vi "Format to Internal Technique Parameters.vi"(8 "error in (no error)":errorcluster, 9 "Technique Parameters (Typedefs)":variant, 10 "Technique":T1, 11 "Potentiostat Galvanostat in":refnum<class "Potentiostat Galvanostat.lvclass">) -> (0 "error out":errorcluster, 2 "Internal Technique Parameters":variant, 3 "Potentiostat Galvanostat out":refnum<class "Potentiostat Galvanostat.lvclass">)   [LabVIEW 2018, in "Potentiostat Galvanostat.lvclass"]
uses:
  Potentiostat Galvanostat.lvclass
  Controls/Technique List.ctl
  Controls/Error Codes.ctl
  Potentiostat Galvanostat.lvclass/Potentiostat Galvanostat.ctl
  Controls/OCV Parameters.ctl
  Controls/OCV Internal Parameters.ctl
  Controls/CV Parameters.ctl
  Controls/CV Internal Parameters.ctl
  Controls/CA Parameters.ctl
  Controls/CA Internal Parameters.ctl
  Controls/CP Parameters.ctl
  Controls/CP Internal Parameters.ctl
  Controls/PEIS Parameters.ctl
  Controls/PEIS Internal Parameters.ctl
  Controls/GEIS Parameters.ctl
  Controls/GEIS Internal Parameters.ctl
  BL_GetErrorMsg.vi
  <vilib>/Utility/error.llb/Error Cluster From Error Code.vi
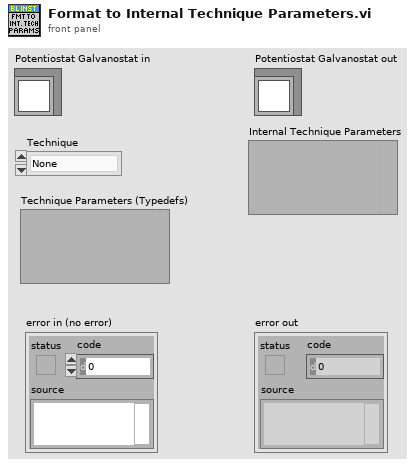
[diagram p1: front panel]
types:
  T1 = typedef "Potentiostat Galvanostat.lvclass/Technique List.ctl" = enum16{"None", "ocv", "cv", "biovscan", "ca", "cp", "iscan", "vscan", "lasv", "load", "pow", "peis", "geis", "seisp", "seisg", "dpv", "swv", "npv", "mpv", "dnpv", "dpa", "evt", "lp", "gc", "cpp", "pdp", "psp", "zra", "ircmp", "pzir", "gzir", "loop", "TO", "TI", "TOS", "vscanlimit", "iscanlimit", "mp", "casp", "casg", "calimit", "cplimit"}
  T2 = typedef "Potentiostat Galvanostat.lvclass/OCV Parameters.ctl" = cluster{"Rest duration (s)":sgl, "Record every dE (V)":sgl, "Record every dT (s)":sgl, "Ewe range":u16, "CE to ground Mode":u16}
  T3 = typedef "Potentiostat Galvanostat.lvclass/OCV Internal Parameters.ctl" = cluster{"Rest_time_T":sgl, "Record_every_dE":sgl, "Record_every_dT":sgl, "E_Range":u16, "em":u16, "ce":u16, "tb":sgl}
  T4 = typedef "Potentiostat Galvanostat.lvclass/CV Parameters.ctl" = cluster{"Ei Params":cluster{"Current step vs initial one (Ei)":bool, "Voltage step (V) (Ei)":sgl, "slew rate array (mV/s) (Ei)":sgl}, "E1 Params":cluster{"Current step vs initial one (E1)":bool, "Voltage step (V) (E1)":sgl, "slew rate array (mV/s) (E1)":sgl}, "E2 Params":cluster{"Current step vs initial one (E2)":bool, "Voltage step (V) (E2)":sgl, "slew rate array (mV/s) (E2)":sgl}, "Ef Params":cluster{"Current step vs initial one (Ef)":bool, "Voltage step (V) (Ef)":sgl, "slew rate array (mV/s) (Ef)":sgl}, "Number of cycle":i32, "recording on dE (V)":sgl, "average every dE":bool, "Begin step accumulation (1 = 100% of step)":sgl, "End step accumulation ( 1 = 100% of step)":sgl, "I range":u16, "Bandwidth":u16, "Ewe range":u16, "CE to ground Mode":u16}
  T5 = typedef "Potentiostat Galvanostat.lvclass/CV Internal Parameters.ctl" = cluster{"Voltage_steps":cluster{"vs_initial":bool, "Voltage_step":sgl, "Scan_Rate":sgl}[], "N_Cycles":i32, "Record_every_dE":sgl, "Average_over_dE":bool, "Begin_measuring_I":sgl, "End_measuring_I":sgl, "I_Range":u16, "E_Range":u16, "Bandwidth":u16, "em":u16, "ce":u16, "Scan_number":u16, "tb":sgl}
  T6 = typedef "Potentiostat Galvanostat.lvclass/CA Parameters.ctl" = cluster{"Voltage Steps":cluster{"Voltage step vs initial one":bool, "Voltage step (V)":sgl, "Duration step (s)":sgl}[], "No. of steps":i32, "Record every dt (s)":sgl, "Record every dI (A)":sgl, "No. of times\ntechnique is repeated":i32, "I range":u16, "Ewe range":u16, "Bandwidth":u16, "CE to ground Mode":u16}
  T7 = typedef "Potentiostat Galvanostat.lvclass/CA Internal Parameters.ctl" = cluster{"tb":sgl, "Voltage_steps":cluster{"vs_initial":bool, "Voltage_step":sgl, "Duration_step":sgl}[], "Step_number":i32, "N_Cycles":i32, "Record_every_dI":sgl, "Record_every_dT":sgl, "I_Range":u16, "E_Range":u16, "Bandwidth":u16, "em":u16, "ce":u16}
  T8 = typedef "Potentiostat Galvanostat.lvclass/CP Parameters.ctl" = cluster{"Current Steps":cluster{"Current step vs initial\none":bool, "Current step (A)":sgl, "Duration step (s)":sgl}[], "No. of steps":i32, "Record every dt (s)":sgl, "Record every dE (V)":sgl, "No. of times\ntechnique is repeated":i32, "I range":u16, "Ewe range":u16, "Bandwidth":u16, "CE to ground Mode":u16}
  T9 = typedef "Potentiostat Galvanostat.lvclass/CP Internal Parameters.ctl" = cluster{"Current_steps":cluster{"vs_initial":bool, "Current_step":sgl, "Duration_step":sgl}[], "Step_number":i32, "N_Cycles":i32, "Record_every_dE":sgl, "Record_every_dT":sgl, "I_Range":u16, "E_Range":u16, "Bandwidth":u16, "em":u16, "ce":u16, "tb":sgl}
  T10 = typedef "Potentiostat Galvanostat.lvclass/PEIS Parameters.ctl" = cluster{"Step duration (s)":sgl, "Record every dI (A)":sgl, "Record every dt (s)":sgl, "Initial voltage step (V)":sgl, "Voltage step vs initial one":bool, "Initial frequency (Hz)":sgl, "sweep linear/logarithmic":bool, "Number of frequencies":i32, "Final frequency (Hz)":sgl, "Sine amplitude (V)":sgl, "No. of repeat times":i32, "No. of period to wait\nbefore each frequency":sgl, "Non-stationary correction":bool, "I Range":u16, "Bandwidth":u16, "CE to ground Mode":u16}
  T11 = typedef "Potentiostat Galvanostat.lvclass/PEIS Internal Parameters.ctl" = cluster{"Step_number":i32, "Initial_Voltage_step":sgl, "vs_initial":bool, "Final_Voltage_step":sgl, "vs_final":bool, "Duration_step":sgl, "Record_every_dI":sgl, "Record_every_dT":sgl, "Initial_frequency":sgl, "sweep":bool, "Final_frequency":sgl, "Frequency_number":i32, "Amplitude_Voltage":sgl, "Wait_for_steady":sgl, "Average_N_times":i32, "Correction":bool, "I_Range":u16, "Bandwidth":u16, "em":u16, "ce":u16}
  T12 = typedef "Potentiostat Galvanostat.lvclass/GEIS Parameters.ctl" = cluster{"Initial frequency (Hz)":sgl, "sweep linear/logarithmic":bool, "Number of frequencies":i32, "Final frequency (Hz)":sgl, "Sine amplitude (A)":sgl, "No. of repeat times":i32, "No. of period to wait\nbefore each frequency":sgl, "Non-stationary correction":bool, "I Range":u16, "Bandwidth":u16, "CE to ground Mode":u16, "Step duration (s)":sgl, "Record every dE (V)":sgl, "Record every dt (s)":sgl, "Initial current step (A)":sgl, "Current step vs initial one":bool}
  T13 = typedef "Potentiostat Galvanostat.lvclass/GEIS Internal Parameters.ctl" = cluster{"Step_number":i32, "Initial_Current_step":sgl, "vs_initial ":bool, "Final_Current_step":sgl, "vs_final":bool, "Duration_step":sgl, "Record_every_dE":sgl, "Record_every_dT":sgl, "Initial_frequency":sgl, "sweep":bool, "Final_frequency":sgl, "Frequency_number":i32, "Amplitude_Current":sgl, "Wait_for_steady":sgl, "Average_N_times":i32, "Correction":bool, "I_Range":u16, "Bandwidth":u16, "em":u16, "ce":u16}
  T14 = typedef "Potentiostat Galvanostat.lvclass/Error Codes.ctl" = i32
  T15 = cluster{"Current step vs initial one (Ei)":bool, "Voltage step (V) (Ei)":sgl, "slew rate array (mV/s) (Ei)":sgl}
  T16 = cluster{"Current step vs initial one (E1)":bool, "Voltage step (V) (E1)":sgl, "slew rate array (mV/s) (E1)":sgl}
  T17 = cluster{"Current step vs initial one (E2)":bool, "Voltage step (V) (E2)":sgl, "slew rate array (mV/s) (E2)":sgl}
  T18 = cluster{"Current step vs initial one (Ef)":bool, "Voltage step (V) (Ef)":sgl, "slew rate array (mV/s) (Ef)":sgl}
  T19 = cluster{"Current step vs initial one (Ef)":bool, "Voltage step (V) (Ef)":sgl, "slew rate array (mV/s) (Ef)":sgl}[]
  T20 = cluster{"Voltage step vs initial one":bool, "Voltage step (V)":sgl, "Duration step (s)":sgl}[]
  T21 = cluster{"Current step vs initial\none":bool, "Current step (A)":sgl, "Duration step (s)":sgl}[]
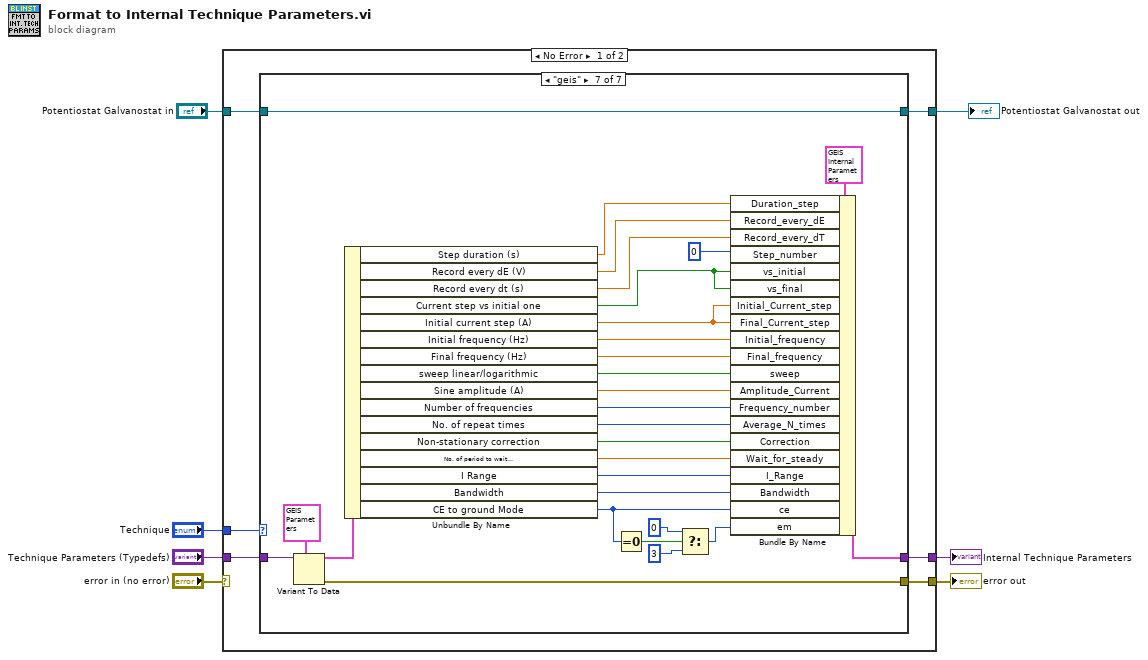
[diagram p0: block diagram]
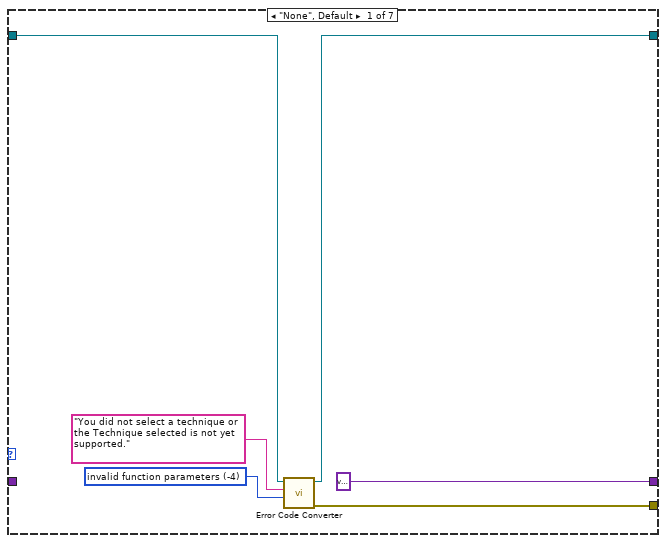
[diagram p2: hidden frame]
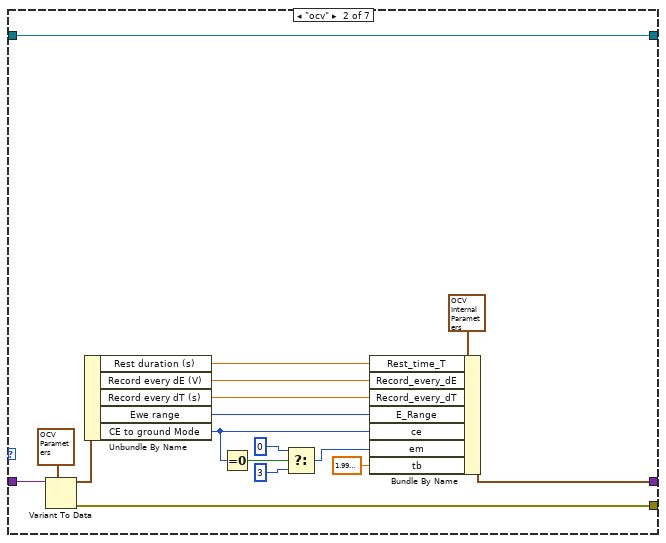
[diagram p3: hidden frame]
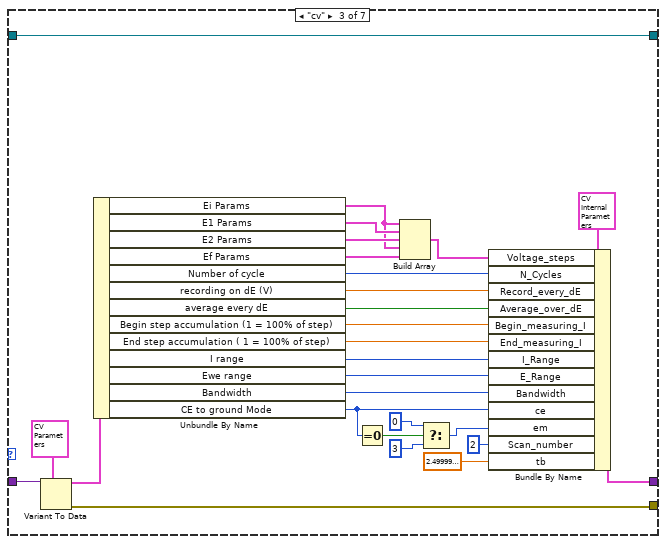
[diagram p4: hidden frame]
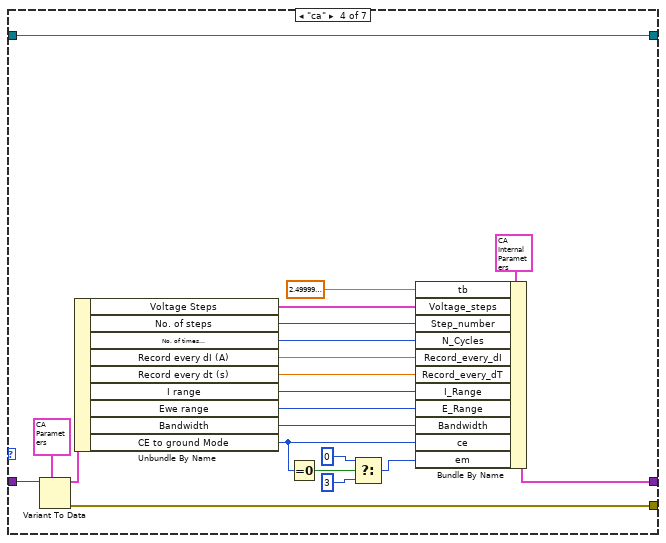
[diagram p5: hidden frame]
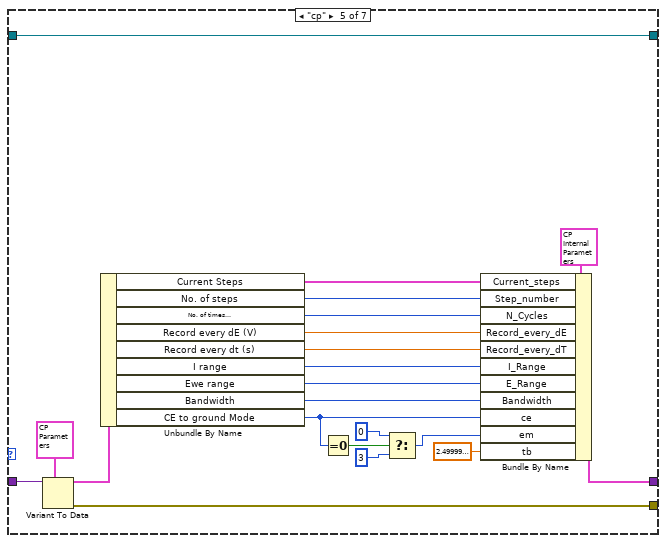
[diagram p6: hidden frame]
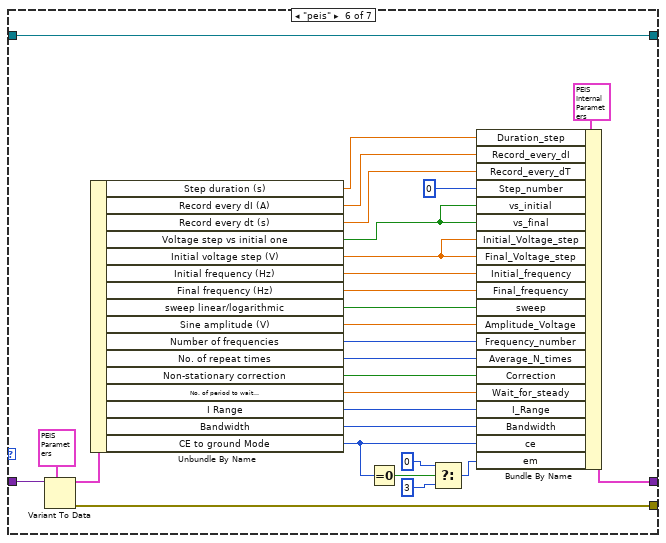
[diagram p7: hidden frame]
diagram:
  n1 = case shown="No Error" "error in (no error)" {
    selector: "error in (no error)" -> [_ w163]
    tunnel: "Technique" -> [w13 _]
    tunnel: "Technique Parameters (Typedefs)" -> [w12 _]
    tunnel: "Potentiostat Galvanostat in" -> [w11 w162]
    tunnel: [w10 w162] -> w4
    tunnel: [w9 w163] -> w3
    tunnel: [w8 _] -> w1
    frame No Error {
      n2 = case shown="\"geis\"" w13 {
        tunnel: w12 -> [_ w23 w39 w68 w87 w114 w141]
        tunnel: w11 -> [w17 w20 w63 w66 w105 w133 w161]
        tunnel: [w16 w20 w63 w66 w105 w133 w161] -> w10
        tunnel: [w14 w22 w38 w65 w86 w113 w140] -> w9
        tunnel: [variant ("Variant") w21 w37 w64 w85 w112 w139] -> w8
        frame "None", Default {
          w19 = T14 -4 items=["No Error"=0, "no instrument connected"=-1, "connection in progress"=-2, "selected channel(s) unplugged"=-3, "invalid function parameters"=-4, "selected file does not exist"=-5, "function failed"=-6, "no channel selected"=-7, "invalid instrument configuration"=-8, "EC-Lab firmware loaded on the instrument"=-9, "library not correctly loaded in memory"=-10, "USB library not correctly loaded in memory"=-11, "function of the library already in progress"=-12, "selected channel(s) already used"=-13, "device not allowed"=-14, "Invalid update function parameters"=-15, "internal instrument communication failed"=-101, "too many data to transfer from the instrument (device error)"=-102, "selected channel(s) unplugged (device error)"=-103, "instrument response error"=-104, "invalid message size"=-105] ("Error Code")
          n3 = call "Error Code Converter.vi"("Error Code"=w19, "Additional Description"="You did not select a technique or the Technique selected is not yet supported.", "Potentiostat Galvanostat in"=w17) -> ("error out"=w14:errorcluster, "Potentiostat Galvanostat out"=w16:refnum<class "Potentiostat Galvanostat.lvclass">)  [unwired: 7 in]
        }
        frame "ocv" {
          n4 = Variant To Data(type=T2 {"Rest duration (s)"=1.0, "Record every dE (V)"=0.01, "Record every dT (s)"=0.01, "Ewe range"=3, "CE to ground Mode"=0} ("OCV Parameters"), Variant=w23) -> (data=w25:T2, error out=w22:errorcluster)  [unwired: 1 in]
          n5 = Unbundle By Name(w25) -> ("Rest duration (s)"=w35:sgl, "Record every dE (V)"=w34:sgl, "Record every dT (s)"=w33:sgl, "Ewe range"=w32:u16, "CE to ground Mode"=w27:u16)
          n6 = Equal To 0?(x=w27) -> (x = 0?=w30:bool)
          n7 = Select(t=u16 0, s=w30, f=u16 3) -> (s? t:f=w26:u16)
          n8 = Bundle By Name(cluster=T3 {"Rest_time_T"=1.0, "Record_every_dE"=0.01, "Record_every_dT"=0.01, "E_Range"=3, "em"=1, "ce"=0, "tb"=2e-05} ("OCV Parameters"), "Rest_time_T"=w35, "Record_every_dE"=w34, "Record_every_dT"=w33, "E_Range"=w32, "ce"=w27, "em"=w26, "tb"=sgl 2e-05) -> (w21:T3)
        }
        frame "cv" {
          n9 = Variant To Data(type=T4 {"Ei Params"={"Current step vs initial one (Ei)"=TRUE, "Voltage step (V) (Ei)"=0.0, "slew rate array (mV/s) (Ei)"=0.1}, "E1 Params"={"Current step vs initial one (E1)"=FALSE, "Voltage step (V) (E1)"=0.1, "slew rate array (mV/s) (E1)"=0.1}, "E2 Params"={"Current step vs initial one (E2)"=FALSE, "Voltage step (V) (E2)"=-0.2, "slew rate array (mV/s) (E2)"=0.1}, "Ef Params"={"Current step vs initial one (Ef)"=TRUE, "Voltage step (V) (Ef)"=0.0, "slew rate array (mV/s) (Ef)"=0.1}, "Number of cycle"=1, "recording on dE (V)"=0.01, "average every dE"=TRUE, "Begin step accumulation (1 = 100% of step)"=0.5, "End step accumulation ( 1 = 100% of step)"=0.75, "I range"=12, "Bandwidth"=5, "Ewe range"=3, "CE to ground Mode"=0} ("CV Parameters"), Variant=w39) -> (data=w40:T4, error out=w38:errorcluster)  [unwired: 1 in]
          n10 = Unbundle By Name(w40) -> ("Ei Params"=w45:T15, "E1 Params"=w47:T16, "E2 Params"=w46:T17, "Ef Params"=w44:T18, "Number of cycle"=w61:i32, "recording on dE (V)"=w60:sgl, "average every dE"=w59:bool, "Begin step accumulation (1 = 100% of step)"=w58:sgl, "End step accumulation ( 1 = 100% of step)"=w57:sgl, "I range"=w56:u16, "Ewe range"=w55:u16, "Bandwidth"=w54:u16, "CE to ground Mode"=w50:u16)
          n11 = Equal To 0?(x=w50) -> (x = 0?=w53:bool)
          n12 = Build Array(w45, w47, w46, w45, w44) -> (w43:T19)
          n13 = Select(t=u16 0, s=w53, f=u16 3) -> (s? t:f=w49:u16)
          n14 = Bundle By Name(cluster=T5 {"Voltage_steps"=[], "N_Cycles"=1, "Record_every_dE"=0.01, "Average_over_dE"=TRUE, "Begin_measuring_I"=0.5, "End_measuring_I"=0.75, "I_Range"=12, "E_Range"=3, "Bandwidth"=5, "em"=1, "ce"=0, "Scan_number"=2, "tb"=2.5e-05} ("CV Parameters"), "Voltage_steps"=w43, "N_Cycles"=w61, "Record_every_dE"=w60, "Average_over_dE"=w59, "Begin_measuring_I"=w58, "End_measuring_I"=w57, "I_Range"=w56, "E_Range"=w55, "Bandwidth"=w54, "ce"=w50, "em"=w49, "Scan_number"=u16 2, "tb"=sgl 2.5e-05) -> (w37:T5)
        }
        frame "ca" {
          n15 = Variant To Data(type=T6 {"Voltage Steps"=[{"Voltage step vs initial one"=TRUE, "Voltage step (V)"=0.0, "Duration step (s)"=1.0}, {"Voltage step vs initial one"=TRUE, "Voltage step (V)"=0.1, "Duration step (s)"=1.0}, {"Voltage step vs initial one"=TRUE, "Voltage step (V)"=0.2, "Duration step (s)"=1.0}], "No. of steps"=2, "Record every dt (s)"=0.01, "Record every dI (A)"=1e-05, "No. of times\ntechnique is repeated"=0, "I range"=12, "Ewe range"=3, "Bandwidth"=5, "CE to ground Mode"=0} ("CA Parameters"), Variant=w68) -> (data=w67:T6, error out=w65:errorcluster)  [unwired: 1 in]
          n16 = Unbundle By Name(w67) -> ("Voltage Steps"=w81:T20, "No. of steps"=w82:i32, "No. of times\ntechnique is repeated"=w80:i32, "Record every dI (A)"=w79:sgl, "Record every dt (s)"=w78:sgl, "I range"=w75:u16, "Ewe range"=w76:u16, "Bandwidth"=w77:u16, "CE to ground Mode"=w71:u16)
          n17 = Equal To 0?(x=w71) -> (x = 0?=w74:bool)
          n18 = Select(t=u16 0, s=w74, f=u16 3) -> (s? t:f=w70:u16)
          n19 = Bundle By Name(cluster=T7 {"tb"=2.5e-05, "Voltage_steps"=[{"vs_initial"=TRUE, "Voltage_step"=0.0, "Duration_step"=1.0}, {"vs_initial"=TRUE, "Voltage_step"=0.1, "Duration_step"=1.0}, {"vs_initial"=TRUE, "Voltage_step"=0.2, "Duration_step"=1.0}], "Step_number"=2, "N_Cycles"=0, "Record_every_dI"=1e-05, "Record_every_dT"=0.01, "I_Range"=8, "E_Range"=3, "Bandwidth"=5, "em"=1, "ce"=0} ("CA Internal Parameters"), "tb"=sgl 2.5e-05, "Voltage_steps"=w81, "Step_number"=w82, "N_Cycles"=w80, "Record_every_dI"=w79, "Record_every_dT"=w78, "I_Range"=w75, "E_Range"=w76, "Bandwidth"=w77, "ce"=w71, "em"=w70) -> (w64:T7)
        }
        frame "cp" {
          n20 = Variant To Data(type=T8 {"Current Steps"=[{"Current step vs initial\none"=FALSE, "Current step (A)"=0.0, "Duration step (s)"=1.0}, {"Current step vs initial\none"=FALSE, "Current step (A)"=0.001, "Duration step (s)"=1.0}, {"Current step vs initial\none"=FALSE, "Current step (A)"=0.005, "Duration step (s)"=1.0}], "No. of steps"=2, "Record every dt (s)"=0.05, "Record every dE (V)"=0.005, "No. of times\ntechnique is repeated"=0, "I range"=8, "Ewe range"=3, "Bandwidth"=5, "CE to ground Mode"=0} ("CP Parameters"), Variant=w87) -> (data=w88:T8, error out=w86:errorcluster)  [unwired: 1 in]
          n21 = Unbundle By Name(w88) -> ("Current Steps"=w104:T21, "No. of steps"=w103:i32, "No. of times\ntechnique is repeated"=w102:i32, "Record every dE (V)"=w100:sgl, "Record every dt (s)"=w101:sgl, "I range"=w99:u16, "Ewe range"=w98:u16, "Bandwidth"=w97:u16, "CE to ground Mode"=w91:u16)
          n22 = Equal To 0?(x=w91) -> (x = 0?=w94:bool)
          n23 = Select(t=u16 0, s=w94, f=u16 3) -> (s? t:f=w90:u16)
          n24 = Bundle By Name(cluster=T9 {"Current_steps"=[{"vs_initial"=FALSE, "Current_step"=0.0, "Duration_step"=1.0}, {"vs_initial"=FALSE, "Current_step"=0.001, "Duration_step"=1.0}, {"vs_initial"=FALSE, "Current_step"=0.005, "Duration_step"=1.0}], "Step_number"=2, "N_Cycles"=0, "Record_every_dE"=0.005, "Record_every_dT"=0.05, "I_Range"=8, "E_Range"=3, "Bandwidth"=5, "em"=1, "ce"=0, "tb"=2.5e-05} ("CP Parameters"), "Current_steps"=w104, "Step_number"=w103, "N_Cycles"=w102, "Record_every_dE"=w100, "Record_every_dT"=w101, "I_Range"=w99, "E_Range"=w98, "Bandwidth"=w97, "ce"=w91, "em"=w90, "tb"=sgl 2.5e-05) -> (w85:T9)
        }
        frame "peis" {
          n25 = Variant To Data(type=T10 {"Step duration (s)"=1.0, "Record every dI (A)"=0.1, "Record every dt (s)"=0.1, "Initial voltage step (V)"=0.0, "Voltage step vs initial one"=TRUE, "Initial frequency (Hz)"=0.0, "sweep linear/logarithmic"=TRUE, "Number of frequencies"=51, "Final frequency (Hz)"=1.0, "Sine amplitude (V)"=0.01, "No. of repeat times"=1, "No. of period to wait\nbefore each frequency"=2.0, "Non-stationary correction"=TRUE, "I Range"=12, "Bandwidth"=5, "CE to ground Mode"=0} ("PEIS Parameters"), Variant=w114) -> (data=w115:T10, error out=w113:errorcluster)  [unwired: 1 in]
          n26 = Unbundle By Name(w115) -> ("Step duration (s)"=w111:sgl, "Record every dI (A)"=w110:sgl, "Record every dt (s)"=w109:sgl, "Voltage step vs initial one"=w108:bool, "Initial voltage step (V)"=w106:sgl, "Initial frequency (Hz)"=w107:sgl, "Final frequency (Hz)"=w132:sgl, "sweep linear/logarithmic"=w131:bool, "Sine amplitude (V)"=w130:sgl, "Number of frequencies"=w129:i32, "No. of repeat times"=w128:i32, "Non-stationary correction"=w127:bool, "No. of period to wait\nbefore each frequency"=w126:sgl, "I Range"=w125:u16, "Bandwidth"=w124:u16, "CE to ground Mode"=w118:u16)
          n27 = Equal To 0?(x=w118) -> (x = 0?=w121:bool)
          n28 = Select(t=u16 0, s=w121, f=u16 3) -> (s? t:f=w117:u16)
          n29 = Bundle By Name(cluster=T11 {"Step_number"=0, "Initial_Voltage_step"=0.0, "vs_initial"=TRUE, "Final_Voltage_step"=1.0, "vs_final"=FALSE, "Duration_step"=1.0, "Record_every_dI"=0.1, "Record_every_dT"=0.1, "Initial_frequency"=100000.0, "sweep"=FALSE, "Final_frequency"=1.0, "Frequency_number"=51, "Amplitude_Voltage"=0.01, "Wait_for_steady"=2.0, "Average_N_times"=1, "Correction"=TRUE, "I_Range"=12, "Bandwidth"=5, "em"=1, "ce"=0} ("PEIS Parameters"), "Duration_step"=w111, "Record_every_dI"=w110, "Record_every_dT"=w109, "Step_number"=0, "vs_initial"=w108, "vs_final"=w108, "Initial_Voltage_step"=w106, "Final_Voltage_step"=w106, "Initial_frequency"=w107, "Final_frequency"=w132, "sweep"=w131, "Amplitude_Voltage"=w130, "Frequency_number"=w129, "Average_N_times"=w128, "Correction"=w127, "Wait_for_steady"=w126, "I_Range"=w125, "Bandwidth"=w124, "ce"=w118, "em"=w117) -> (w112:T11)
        }
        frame "geis" {
          n30 = Variant To Data(type=T12 {"Initial frequency (Hz)"=100000.0, "sweep linear/logarithmic"=FALSE, "Number of frequencies"=51, "Final frequency (Hz)"=1.0, "Sine amplitude (A)"=0.001, "No. of repeat times"=1, "No. of period to wait\nbefore each frequency"=2.0, "Non-stationary correction"=TRUE, "I Range"=12, "Bandwidth"=5, "CE to ground Mode"=0, "Step duration (s)"=1.0, "Record every dE (V)"=0.1, "Record every dt (s)"=0.1, "Initial current step (A)"=0.0, "Current step vs initial one"=TRUE} ("GEIS Parameters"), Variant=w141) -> (data=w143:T12, error out=w140:errorcluster)  [unwired: 1 in]
          n31 = Unbundle By Name(w143) -> ("Step duration (s)"=w138:sgl, "Record every dE (V)"=w137:sgl, "Record every dt (s)"=w136:sgl, "Current step vs initial one"=w135:bool, "Initial current step (A)"=w134:sgl, "Initial frequency (Hz)"=w155:sgl, "Final frequency (Hz)"=w154:sgl, "sweep linear/logarithmic"=w153:bool, "Sine amplitude (A)"=w152:sgl, "Number of frequencies"=w151:i32, "No. of repeat times"=w150:i32, "Non-stationary correction"=w149:bool, "No. of period to wait\nbefore each frequency"=w148:sgl, "I Range"=w147:u16, "Bandwidth"=w146:u16, "CE to ground Mode"=w145:u16)
          n32 = Equal To 0?(x=w145) -> (x = 0?=w159:bool)
          n33 = Select(t=u16 0, s=w159, f=u16 3) -> (s? t:f=w156:u16)
          n34 = Bundle By Name(cluster=T13 {"Step_number"=0, "Initial_Current_step"=0.0, "vs_initial "=TRUE, "Final_Current_step"=0.001, "vs_final"=TRUE, "Duration_step"=1.0, "Record_every_dE"=0.1, "Record_every_dT"=0.1, "Initial_frequency"=100000.0, "sweep"=FALSE, "Final_frequency"=1.0, "Frequency_number"=51, "Amplitude_Current"=0.001, "Wait_for_steady"=2.0, "Average_N_times"=1, "Correction"=TRUE, "I_Range"=7, "Bandwidth"=5, "em"=1, "ce"=0} ("GEIS Parameters"), "Duration_step"=w138, "Record_every_dE"=w137, "Record_every_dT"=w136, "Step_number"=0, "vs_initial"=w135, "vs_final"=w135, "Initial_Current_step"=w134, "Final_Current_step"=w134, "Initial_frequency"=w155, "Final_frequency"=w154, "sweep"=w153, "Amplitude_Current"=w152, "Frequency_number"=w151, "Average_N_times"=w150, "Correction"=w149, "Wait_for_steady"=w148, "I_Range"=w147, "Bandwidth"=w146, "ce"=w145, "em"=w156) -> (w139:T13)
        }
      }
    }
    frame Error {
    }
  }
  "error out" <- w3
  "Potentiostat Galvanostat out" <- w4
  "Internal Technique Parameters" <- w1
